vi "SelectSlide.vi"() -> (0 "Success":bool, 1 "names":string[](array[string]))   [LabVIEW 2012]
uses:
  SlideParams.ctl
panel:
  out "Slide":picture
  in  "Available Slides":i32[](listbox)
  in  "Cancel":bool
  in  "Ok":bool
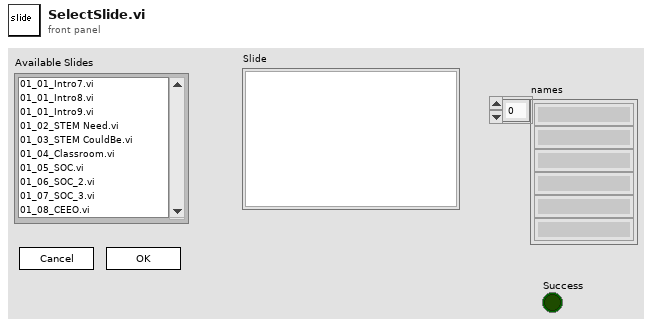
[diagram p1: front panel]
types:
  T1 = typedef "SlideParams.ctl" = enum32{"No Selection", "Bounce", "Order", "Hide", "Remove"}
  T2 = typedef "LVBoundsTypeDef.ctl" = cluster{"Width":u32, "Height":u32}
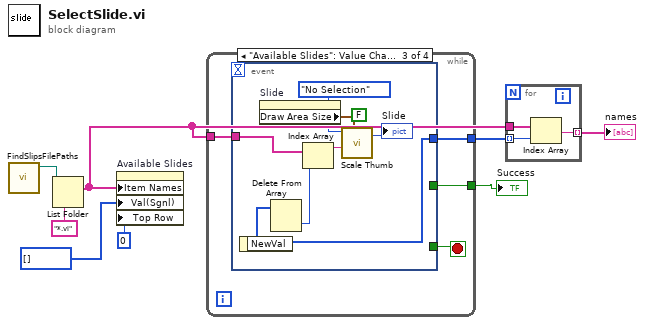
[diagram p0: block diagram]
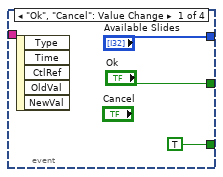
[diagram p2: hidden frame]
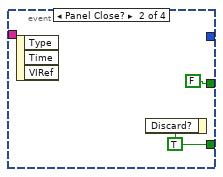
[diagram p3: hidden frame]
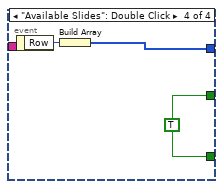
[diagram p4: hidden frame]
diagram:
  n1 = call "FindSlipsFilePaths.vi"() -> ("Slides"=w7:path)  [unwired: 2 in, 4 out]
  n2 = List Folder(path=w7, pattern="*.vi") -> (filenames=w4:string[])  [unwired: 2 in, 3 out]
  n3 = property on="Available Slides" class="LstBox (strict)"("Item Names"=w4, "Val(Sgnl)"=i32[] [], "Top Row"=0 ("Available Templates")) -> ()  [unwired: 2 in, 2 out]
  n4 = while {
    tunnel: [w11] -> w6
    tunnel: [w10] -> w5
    tunnel: w4 -> [w9]
    stop <- w12 stop-if-true
    n5 = event shown="[2] \"Available Slides\": Value Change" {
      selector: _ -> [_ _ _ _]
      dyn-events: _ -> [_ _ _ _]
      timeout: _ -> [_ _ _ _]
      tunnel: [TRUE w17 _ w28] -> w12
      tunnel: ["Ok" FALSE _ w28] -> w11
      tunnel: ["Available Slides" _ w20 w26] -> w10
      tunnel: w9 -> [_ _ w25 _]
      event "Ok", "Cancel": Value Change {
        n6 = event-data() -> ()  [unwired: 1 in, 5 out]
      }
      event Panel Close? {
        w17 = TRUE
        n7 = event-data() -> ()  [unwired: 1 in, 3 out]
        n8 = event-data("Discard?"=w17) -> ()  [unwired: 1 in, 1 out]
      }
      event "Available Slides": Value Change {
        n9 = event-data() -> ("NewVal"=w20:i32[])  [unwired: 1 in]
        n10 = property on="Slide" class="Pict"() -> ("Draw Area Size"=w22:T2)  [unwired: 2 in, 2 out]
        n11 = Delete From Array(array=w20) -> (deleted portion=w18:i32)  [unwired: 2 in, 1 out]
        n12 = Index Array(array=w25, index=w18) -> (element=w24:string)
        n13 = call "Scale Thumb.vi"("Desired Dimensions"=w22, "Full Size"=FALSE ("Show Labels"), "file"=w24, "Mod"=SlideParams."No Selection") -> ("new picture"=→"Slide":picture)  [unwired: 2 in, 1 out]
      }
      event "Available Slides": Double Click {
        w28 = TRUE
        n14 = event-data() -> ("Row"=w27:i32)  [unwired: 1 in]
        n15 = Build Array(w27) -> (w26:i32[])
      }
    }
  }
  "Success" <- w6
  n16 = for {
    tunnel: [w31] -> w1 mode=indexing
    tunnel: w5 -> [w30] mode=indexing
    tunnel: w4 -> [w29]
    n17 = Index Array(array=w29, index=w30) -> (element=w31:string)
  }
  "names" <- w1
